vi "Init.vi"(8 "error in (no error)":errorcluster, 11 "Data in":refnum<class "DAQmx - Analog Output Multi Sample.lvclass">) -> (0 "error out":errorcluster, 3 "Data out":refnum<class "DAQmx - Analog Output Multi Sample.lvclass">)   [LabVIEW 2021, in "DAQmx - Analog Output Multi Sample.lvclass"]
doc: "Abstract Data Classes 2.1.1.13\nTim Streeter - TSA\nCopyright (c) 2025, TSA"
uses:
  DAQmx - Analog Output Multi Sample.lvclass
  C:/Program Files (x86)/National Instruments/LabVIEW 2021/vi.lib/TSA/Omni-Bus/Omni-Bus/Bus Access/Bus_Access.lvclass
  C:/TSA/DAQmx-Bus/Source/DAQmx-Bus.lvclass
  <vilib>/TSA/Omni-Bus/Omni-Bus/Bus Access/Bus_Access.lvclass/Bus_Access.ctl
  DAQmx - Analog Output Multi Sample.lvclass/DAQmx - Analog Output Multi Sample.ctl
  Types/Waveform/DAQmx-Bus_Waveform_Type.lvclass
  C:/Program Files (x86)/National Instruments/LabVIEW 2021/vi.lib/TSA/Abstract Data Classes/Abs_Types/Value/Abs_Value.lvclass
  C:/Program Files (x86)/National Instruments/LabVIEW 2021/vi.lib/TSA/Abstract Data Classes/Abs_Types/Type/Abs_Type.lvclass
  Types/Waveform/DAQmx-Bus_Waveform_Type.lvclass/DAQmx-Bus_Waveform_Type.ctl
  DAQmx-Bus.lvclass/DAQmx-Bus.ctl
  Types/Waveform/Properties/Write Values DVR.vi
  Types/Waveform/Properties/Write Index.vi
  <vilib>/TSA/Omni-Bus/Omni-Bus/Bus Access/Properties/Read Tags.vi
  Properties/Write Actor Ref.vi
  <vilib>/TSA/Omni-Bus/Omni-Bus/Bus Access/Properties/Write Values.vi
  Support/Actor.vi
  DAQmx-Bus.lvclass
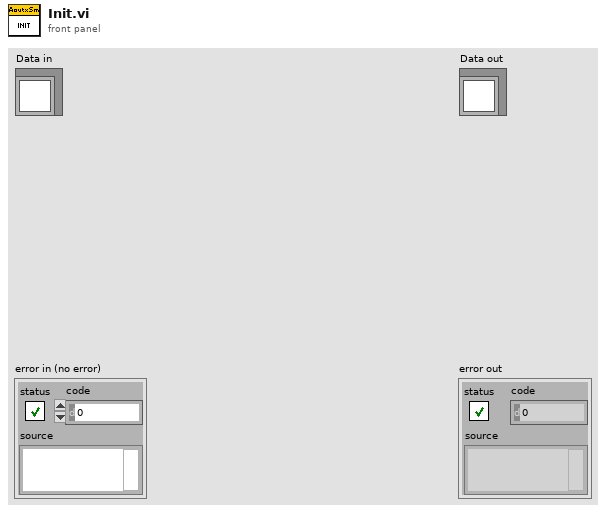
[diagram p1: front panel]
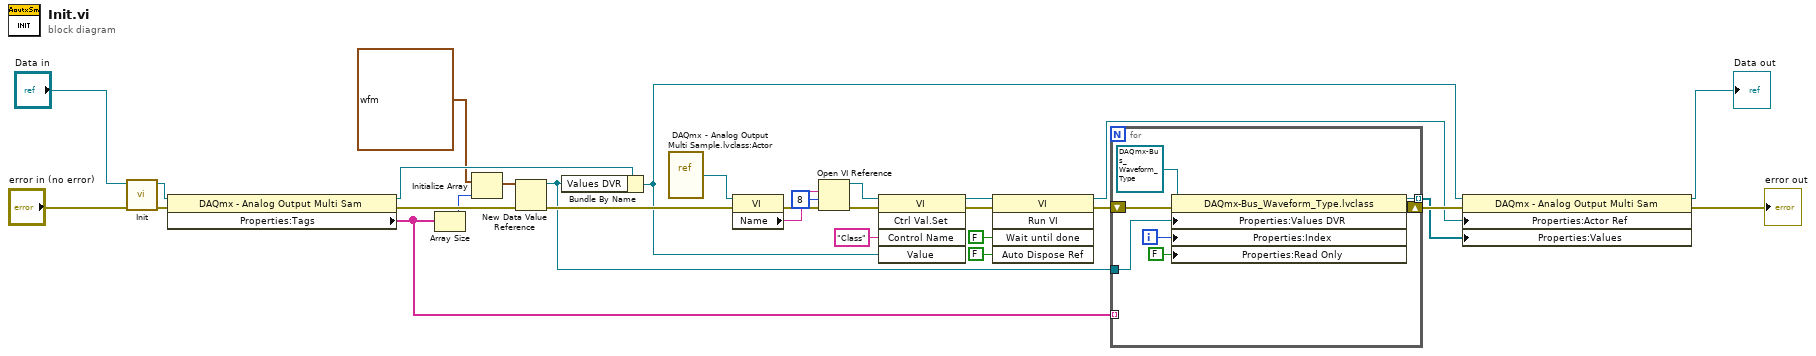
[diagram p0: block diagram]
diagram:
  n1 = call-parent "Init.vi"("error in (no error)"="error in (no error)", "Data in"="Data in") -> ("error out"=w19:errorcluster, "Data out"=w18:refnum<class "DAQmx - Analog Output Multi Sample.lvclass">)  [unwired: 8 in]
  n2 = property class="DAQmx - Analog Output Multi Sam"(reference=w18, error in=w19) -> (reference out=w14:refnum<class "DAQmx - Analog Output Multi Sample.lvclass">, error out=w17:errorcluster, "Properties:Tags"=w12:string[])
  n3 = Array Size(array=w12) -> (size(s)=w16:i32)
  n4 = Initialize Array(waveform(dbl) {"t0"=timestamp(0 s since 1904-01-01), "dt"=1.0, "Y"=[]} ("Waveform"), w16) -> (w15:waveform(dbl)[])
  n5 = New Data Value Reference(data value=w15, error in=w17) -> (data value reference=w10:refnum<data-value>, error out=w28:errorcluster)
  n6 = Bundle By Name(cluster=w14, "Values DVR"=w10) -> (w11:refnum<class "DAQmx - Analog Output Multi Sample.lvclass">)
  n7 = vi-ref "DAQmx - Analog Output Multi Sample.lvclass:Actor.vi"() -> (w27:refnum<vi>)
  n8 = property class="VI"(reference=w27, error in=w28) -> (error out=w25:errorcluster, "Name"=w26:string)  [unwired: 1 out]
  n9 = Open VI Reference(vi path=w26, options=8, error in (no error)=w25) -> (vi reference=w23:refnum<vi>, error out=w24:errorcluster)  [unwired: 3 in]
  n10 = invoke class="VI" method="Ctrl Val.Set"(reference=w23, error in=w24, "Control Name"="Class", "Value"=w11) -> (reference out=w7:refnum<vi>, error out=w6:errorcluster)  [unwired: 1 in, 3 out]
  n11 = invoke class="VI" method="Run VI"(reference=w7, error in=w6, "Wait until done"=FALSE ("Wait Until Done"), "Auto Dispose Ref"=FALSE ("Auto Dispose Reference")) -> (reference out=w4:refnum<vi>, error out=w5:errorcluster)  [unwired: 1 in, 3 out]
  n12 = for {
    shift-right: [w36] -> w13
    shift-left: w5 -> [w37]
    tunnel: w12 -> [_] mode=indexing
    tunnel: w10 -> [w34]
    tunnel: [w33] -> w9 mode=indexing
    i -> [w35]
    n13 = property class="DAQmx-Bus_Waveform_Type.lvclass"(reference=refnum<class "DAQmx-Bus_Waveform_Type.lvclass"> refnum ("DAQmx-Bus_Waveform_Type.lvclass"), error in=w37, "Properties:Values DVR"=w34, "Properties:Index"=w35, "Properties:Read Only"=FALSE ("Read Only")) -> (reference out=w33:refnum<class "DAQmx-Bus_Waveform_Type.lvclass">, error out=w36:errorcluster)
  }
  n14 = property class="DAQmx - Analog Output Multi Sam"(reference=w11, error in=w13, "Properties:Actor Ref"=w4, "Properties:Values"=w9) -> (reference out=→"Data out":refnum<class "DAQmx - Analog Output Multi Sample.lvclass">, error out=→"error out":errorcluster)
